vi "BuildRasterSequence.vi"(7 "RasterDef":T6={"Nyquist, mm"=28.0, "Window, cm"=42.0, "Polarization, V0 H1"=enum."Vertical", "RF Direction Tx0"=enum."Tx - RF In"}, 8 "error in (no error)":errorcluster, 9 "TestZT":cluster{"Z mm":dbl, "Horizontal T deg":dbl}={"Z mm"=0.0, "Horizontal T deg"=1.0}, 10 "Position Array in":T5(array[cluster]), 11 "Sequence in":refnum<class "Sequence.lvclass">) -> (0 "error out":errorcluster, 1 "Raster Sequence":T1[](array[typedef]), 3 "Sequence out":refnum<class "Sequence.lvclass">)   [LabVIEW 2018, in "Sequence.lvclass"]
doc: "This VI builds a sequence for only one RF Direction and one polarization. It is called once. Run multiple directions and polarizations by calling multiple time this from a higher level.\nBuilds a sequence:\nconfig 64 modules\nfor each raster position {\n Motion (X, Y, Z, T Hor)\n Sweep & Log\n}"
uses:
  Sequence.lvclass
  aparCfg/rasterConfig.ctl
  SequenceSubvis/PolarizationSelect.ctl
  SequenceSubvis/RF Direction.ctl
  SequenceSubvis/TestStep-StepType.ctl
  SequenceSubvis/TestStepTypes.ctl
  SequenceSubvis/mWaveTestStep.ctl
  APARMainSubvis/VXM Public API/singleAxisMoveDef.ctl
  APARMainSubvis/VXM Public API/mmWaveAxis.ctl
  Sequence.lvclass/Sequence.ctl
panel:
  out "size(s)":i32
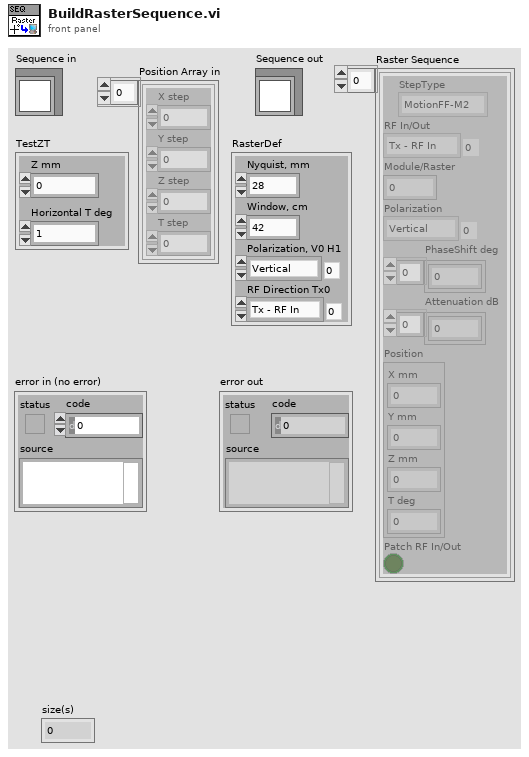
[diagram p1: front panel]
types:
  T1 = typedef "TestStep-StepType.ctl" = cluster{"StepType":T2, "RF In/Out":T3, "Module/Raster":i32, "Polarization":T4, "PhaseShift deg":dbl[], "Attenuation dB":dbl[], "Position":cluster{"X mm":dbl, "Y mm":dbl, "Z mm":dbl, "T deg":dbl}, "Patch RF In/Out":bool}
  T2 = typedef "TestStepTypes.ctl" = enum16{"MotionFF-M2", "Motion", "SweepTest", "RasterTest", "Finish", "64ModuleCfg"}
  T3 = typedef "RF Direction.ctl" = enum16{"Tx - RF In", "Rx - RF Out"}
  T4 = typedef "PolarizationSelect.ctl" = enum16{"Vertical", "Horizontal"}
  T5 = cluster{"X step":dbl, "Y step":dbl, "Z step":dbl, "T step":dbl}[]
  T6 = typedef "rasterConfig.ctl" = cluster{"Nyquist, mm":dbl, "Window, cm":dbl, "Polarization, V0 H1":T4, "RF Direction Tx0":T3}
  T7 = typedef "mWaveTestStep.ctl" = cluster{"StepType":T2, "RF In/Out":T3, "Module/Raster":i32, "Polarization":T4, "AO-64 Array":dbl[], "Position":T8[]}
  T8 = typedef "singleAxisMoveDef.ctl" = cluster{"mmWave Axis":T9, "eng. value":dbl}
  T9 = typedef "mmWaveAxis.ctl" = string
  T10 = cluster{"X mm":dbl, "Y mm":dbl, "Z mm":dbl, "T deg.":dbl}[]
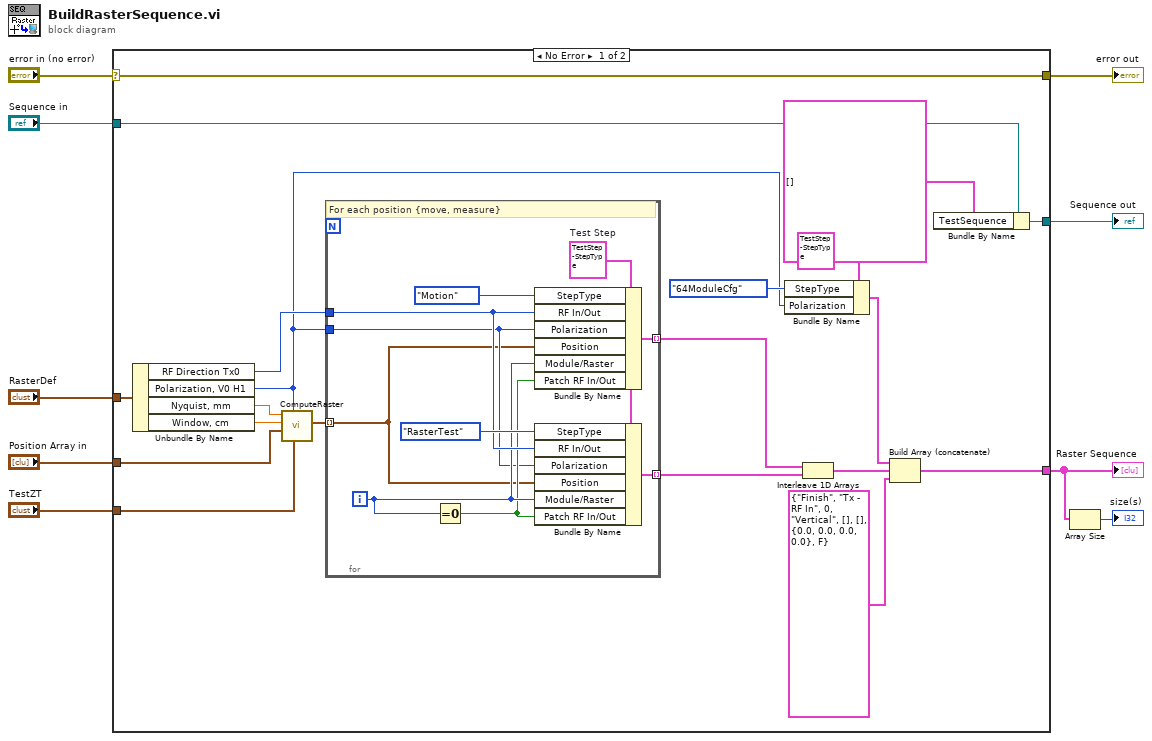
[diagram p0: block diagram]
diagram:
  n1 = case shown="No Error" "error in (no error)" {
    selector: "error in (no error)" -> [w29 w41]
    tunnel: [w29 w41] -> w8
    tunnel: [w17 w40] -> w6
    tunnel: "Sequence in" -> [w18 w40]
    tunnel: "Position Array in" -> [w23 _]
    tunnel: "TestZT" -> [w20 _]
    tunnel: "RasterDef" -> [w19 _]
    tunnel: [w16 _] -> w1
    frame No Error {
      n2 = Unbundle By Name(w19) -> ("RF Direction Tx0"=w12:T3, "Polarization, V0 H1"=w11:T4, "Nyquist, mm"=w21:dbl, "Window, cm"=w22:dbl)
      n3 = call "ComputeRaster.vi"("TestZT"=w20, "Polarization, V0 H1"=w11, "Position Array in"=w23, "Window dimension"=w22, "Nyquist, mm"=w21) -> ("Position Array out"=w24:T10)  [unwired: 3 in, 3 out]
      n4 = for {
        tunnel: w24 -> [w30] mode=indexing
        tunnel: w12 -> [w37]
        tunnel: [w35] -> w26 mode=indexing
        tunnel: [w34] -> w27 mode=indexing
        tunnel: w11 -> [w31]
        i -> [w33]
        w36 = T1 {"StepType"=enum."Motion", "RF In/Out"=enum."Tx - RF In", "Module/Raster"=0, "Polarization"=enum."Horizontal", "PhaseShift deg"=[], "Attenuation dB"=[], "Position"={"X mm"=0.0, "Y mm"=0.0, "Z mm"=0.0, "T deg"=0.0}, "Patch RF In/Out"=FALSE}  # Test Step
        # "For each position {move, measure}"
        n5 = Equal To 0?(x=w33) -> (x = 0?=w32:bool)
        n6 = Bundle By Name(cluster=w36, "StepType"=TestStepTypes."Motion", "RF In/Out"=w37, "Polarization"=w31, "Position"=w30, "Module/Raster"=w33, "Patch RF In/Out"=w32) -> (w35:T1)
        n7 = Bundle By Name(cluster=w36, "StepType"=TestStepTypes."RasterTest", "RF In/Out"=w37, "Polarization"=w31, "Position"=w30, "Module/Raster"=w33, "Patch RF In/Out"=w32) -> (w34:T1)
      }
      n8 = Bundle By Name(cluster=T1 {"StepType"=enum."64ModuleCfg", "RF In/Out"=enum."Tx - RF In", "Module/Raster"=0, "Polarization"=enum."Vertical", "PhaseShift deg"=[], "Attenuation dB"=[], "Position"={"X mm"=0.0, "Y mm"=0.0, "Z mm"=0.0, "T deg"=0.0}, "Patch RF In/Out"=FALSE} ("Test"), "StepType"=TestStepTypes."64ModuleCfg", "Polarization"=w11) -> (w13:T1)
      n9 = Interleave 1D Arrays(w26, w27) -> (w28:T1[])
      n10 = Build Array (concatenate)(w13, w28, T1 {"StepType"=enum."Finish", "RF In/Out"=enum."Tx - RF In", "Module/Raster"=0, "Polarization"=enum."Vertical", "PhaseShift deg"=[], "Attenuation dB"=[], "Position"={"X mm"=0.0, "Y mm"=0.0, "Z mm"=0.0, "T deg"=0.0}, "Patch RF In/Out"=FALSE} ("Test")) -> (w16:T1[])
      n11 = Bundle By Name(cluster=w18, "TestSequence"=T7[] []) -> (w17:refnum<class "Sequence.lvclass">)
    }
    frame Error {
    }
  }
  "error out" <- w8
  "Sequence out" <- w6
  "Raster Sequence" <- w1
  n12 = Array Size(array=w1) -> (size(s)=→"size(s)":i32)
